vi "Create Serial.vi"(4 "Timeout":u32=3000, 5 "Stop Bits":u8=1, 6 "Parity":T1=enum."None", 7 "Data Bits":u8=8, 8 "error in (no error)":errorcluster, 9 "Baudrate":u32=57600, 10 "Serial Port":string) -> (0 "error out":errorcluster, 3 "LINX Server out":refnum<class "LINX Server.lvclass">)   [LabVIEW 2020, in "LINX Server.lvclass"]
uses:
  LINX Server.lvclass
  Typedef/Parity.ctl
  LINX Base.lvclass
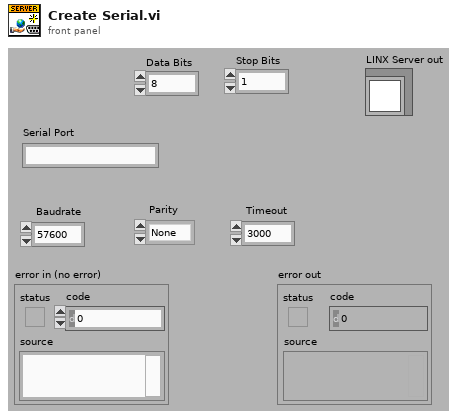
[diagram p1: front panel]
types:
  T1 = typedef "LINX Base.lvclass/Parity.ctl" = enum8{"Invalid", "None", "Odd", "Even", "Mark", "Space"}
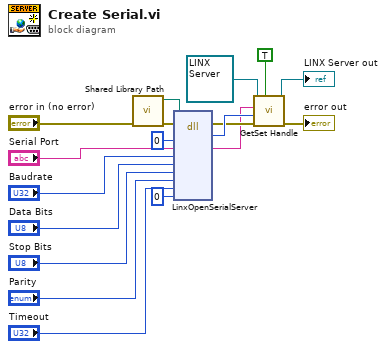
[diagram p0: block diagram]
diagram:
  n1 = call "Shared Library Path.vi"("error in (no error)"="error in (no error)") -> ("error out"=w18:errorcluster, "Path"=w16:path)  [unwired: 9 out]
  n2 = dll-call lib="Z:/Development/LabVIEW Hobbyist Toolkit/LabVIEW/vi.lib/MakerHub/LINX/Resources/libLinxDevice.dll" fn="LinxOpenSerialServer"(path in=w16, error in=w18, "LinxDevice"=u64 0, "name"="Serial Port", "baudrate"="Baudrate", "dataBits"="Data Bits", "stopBits"="Stop Bits", "parity"="Parity", "timeout"="Timeout", "autolaunch"=0) -> (error out=w6:errorcluster, "LinxListener"=w7:u64, "name"=w1:string)  [unwired: 6 in, 3 out]
  n3 = call-dynamic "GetSet Handle.vi"("store (F)"=TRUE, "error in"=w6, "handle in"=w7, "connection"=w1, "LINX Base in"=refnum<class "LINX Server.lvclass"> refnum ("LINX Server out")) -> ("error out"=→"error out":errorcluster, "LINX Base out"=→"LINX Server out":refnum<class "LINX Server.lvclass">)  [unwired: 5 out]
